vi "RayFanModelIntersection.vi"() -> ()   [LabVIEW 2014]
panel:
  in  "Power":dbl=1200.0 format="%#_13g"
  out "Temp":dbl
  in  "Outside":bool
  out "WeldVsRadius":dbl[](graph)=[1.0, 1.0, 1.0, 1.0, 1.0, 1.0, 1.0, 1.0, 1.0, 1.0, 0.958, 0.93, 0.89, 0.876, 0.852, 0.832, 0.814, 0.8, 0.788, 0.77]
  out "BinSize (mm)":dbl=0.05
  in  "NumBins":dbl=20.0
  out "Dists":cluster{dbl[]}[](array[cluster])=[{[]}, {[]}, {[0.558064432912235]}, {[0.7065110965552522]}, {[]}, {[]}, {[]}, {[]}, {[]}, {[]}, {[]}, {[]}, {[]}, {[]}, {[]}, {[0.5450720152295433]}, {[]}, {[]}, {[]}, {[]}, {[0.7012931044326173]}, {[]}, {[]}, {[]}, {[]}, {[]}, {[]}, {[]}, {[0.7332327965683694]}, {[]}, {[]}, {[]}, {[]}, {[0.9493389374686801]}, {[]}, {[]}, {[]}, {[]}, {[]}, {[]}, {[]}, {[0.64928815624828]}, {[]}, {[0.5406762941256205]}, {[]}, {[]}, {[]}, {[]}, {[]}, {[]}, {[]}, {[]}, {[]}, {[0.5086855573476655]}, {[0.5165368704444614]}, {[]}, {[]}, {[0.9647195737987346]}, {[]}, {[]}, {[]}, {[]}, {[0.6161935056556245]}, {[]}, {[]}, {[]}, {[0.6599666981158043]}, {[0.7575878284267049]}, {[]}, {[]}, {[]}, {[0.6345232898235499]}, {[]}, {[]}, {[0.6975266082013275]}, {[]}, {[0.5491594605386263]}, {[0.5884365935336494]}, {[]}, {[]}, {[0.550418714991808]}, {[]}, {[]}, {[]}, {[]}, {[]}, {[]}, {[]}, {[]}, {[0.547517307123691]}, {[]}, {[]}, {[0.9629712723340546]}, {[]}, {[]}, {[]}, {[]}, {[]}, {[0.7196533645578476]}, {[]}, {[]}, {[0.7873333536260919]}, {[0.5571630383766993]}, {[]}, {[]}, {[]}, {[]}, {[]}, {[]}, {[]}, {[]}, {[]}, {[]}, {[]}, {[]}, {[]}, {[]}, {[]}, {[]}, {[]}, {[0.8921440487629841]}, {[]}, {[]}, {[0.5170623590293416]}, {[0.6003465621820364]}, {[]}, {[]}, {[0.7197465893934318]}, {[]}, {[]}, {[]}, {[]}, {[0.6422717159108584]}, {[]}, {[]}, {[]}, {[]}, {[0.8502006061404428]}, {[]}, {[]}, {[]}, {[]}, {[]}, {[]}, {[]}, {[0.8002135268034918]}, {[]}, {[0.9244653981574149]}, {[]}, {[]}, {[]}, {[]}, {[]}, {[]}, {[0.8127103296432845]}, {[0.8494637102867976]}, {[]}, {[0.5768330500604705]}, {[]}, {[]}, {[0.7971462061943174]}, {[0.5190450538376525]}, {[]}, {[]}, {[0.54203797008764]}, {[]}, {[0.8445112253029017]}, {[]}, {[]}, {[]}, {[]}, {[0.6062550701542475]}, {[]}, {[]}, {[]}, {[]}, {[]}, {[0.7489732042547229]}, {[]}, {[0.8330170817130215]}, {[]}, {[]}, {[]}, {[0.5113666314516164]}, {[0.5498423755123026]}, {[0.7182864687625854]}, {[]}, {[]}, {[]}, {[]}, {[0.6517000534238575]}, {[]}, {[]}, {[0.5789678042492773]}, {[]}, {[]}, {[0.8993049672269428]}, {[0.6085788863115259]}, {[]}, {[0.6204881702091252]}, {[0.9649855049671213]}, {[0.660813864499079]}, {[0.9515616425304806]}, {[]}, {[0.8860520397526913]}, {[]}, {[0.97607827123549]}, {[]}, {[]}, {[]}, {[0.7559538054396471]}, {[]}, {[]}, {[0.8221698352656399]}, {[]}, {[]}, {[]}, {[]}, {[]}, {[]}, {[]}, {[0.5536090969205018]}, {[]}, {[]}, {[]}, {[]}, {[]}, {[0.702817978975694]}, {[]}, {[]}, {[0.6470947342089964]}, {[]}, {[]}, {[0.8120625142610847]}, {[0.5281933009897772]}, {[]}, {[]}, {[]}, {[]}, {[]}, {[]}, {[0.5260646334990027]}, {[]}, {[]}, {[]}, {[]}, {[0.5578229776474865]}, {[]}, {[]}, {[]}, {[]}, {[]}, {[]}, {[]}, {[0.6516324141278934]}, {[]}, {[]}, {[]}, {[0.7277751404296459]}, {[]}, {[0.7346441626947963]}, {[]}, {[0.6018486699053848]}, {[]}, {[]}, {[]}, {[]}, {[0.6609968544557817]}, {[]}, {[]}, {[0.8624857635568423]}, {[]}, {[]}, {[]}, {[]}, {[0.5223973616642758]}, {[]}, {[]}, {[]}, {[]}, {[]}, {[]}, {[]}, {[]}, {[0.6499055476854614]}, {[]}, {[]}, {[]}, {[]}, {[]}, {[]}, {[]}, {[]}, {[]}, {[]}, {[]}, {[]}, {[]}, {[]}, {[]}, {[]}, {[]}, {[]}, {[]}, {[]}, {[]}, {[0.9645688700654612]}, {[]}, {[]}, {[]}, {[]}, {[]}, {[0.8409319062965085]}, {[0.5676961462040259]}, {[0.5428966812044365]}, {[]}, {[]}, {[]}, {[]}, {[]}, {[]}, {[]}, {[]}, {[]}, {[]}, {[0.6075630097775284]}, {[0.6825860604163353]}, {[0.5509754449188999]}, {[0.6287420680195404]}, {[]}, {[0.7824466022421895]}, {[]}, {[]}, {[]}, {[]}, {[]}, {[]}, {[]}, {[]}, {[0.92510946600259]}, {[]}, {[]}, {[]}, {[0.8117899400246639]}, {[0.9767679229503767]}, {[]}, {[]}, {[]}, {[]}, {[]}, {[]}, {[]}, {[]}, {[0.7660735839595996]}, {[]}, {[0.7653390306487524]}, {[]}, {[0.6218747267304856]}, {[0.7980078782480812]}, {[]}, {[]}, {[0.6467511427181266]}, {[]}, {[]}, {[]}, {[]}, {[]}, {[]}, {[]}, {[0.961256735044041]}, {[]}, {[0.5285504192342666]}, {[0.7691150491851212]}, {[]}, {[]}, {[]}, {[]}, {[]}, {[]}, {[]}, {[]}, {[]}, {[]}, {[]}, {[]}, {[]}, {[0.6477695496575054]}, {[]}, {[0.5827289010967698]}, {[]}, {[]}, {[]}, {[0.8661418049454438]}, {[]}, {[]}, {[0.9367031742857802]}, {[]}, {[0.5545590410570911]}, {[]}, {[0.5377050699071217]}, {[]}, {[]}, {[0.7438854029234935]}, {[]}, {[]}, {[]}, {[]}, {[]}, {[]}, {[]}, {[]}, {[0.9431758423974651]}, {[]}, {[]}, {[]}, {[]}, {[]}, {[]}, {[]}, {[]}, {[0.6252002539116622]}, {[]}, {[]}, {[]}, {[]}, {[]}, {[]}, {[]}, {[]}, {[]}, {[]}, {[]}, {[0.52847622764937]}, {[0.6440499209435737]}, {[0.5076983622978631]}, {[]}, {[]}, {[]}, {[]}, {[]}, {[]}, {[]}, {[]}, {[]}, {[]}, {[]}, {[]}, {[]}, {[0.5107329517659359]}, {[]}, {[]}, {[]}, {[]}, {[]}, {[]}, {[]}, {[]}, {[]}, {[]}, {[]}, {[]}, {[]}, {[0.8999320044818604]}, {[]}, {[]}, {[]}, {[]}, {[0.524487828892231]}, {[0.6157343526823348]}, {[]}, {[]}, {[]}, {[0.5775248493157631]}, {[0.633099142329562]}, {[]}, {[]}, {[0.9280184819194474]}, {[]}, {[]}, {[]}, {[]}, {[]}, {[]}, {[]}, {[]}, {[]}, {[0.5746835528787432]}, {[]}, {[0.77311121633859]}, {[]}, {[]}, {[]}, {[]}, {[0.7007929147798608]}, {[]}, {[]}, {[]}, {[0.9727918978336536]}, {[]}, {[]}]
  in  "Length":dbl=1.0 format="%#_13g"
  in  "Rays":u32=500
  in  "Point":cluster{"X":dbl, "Y":dbl, "Z":dbl}={"X"=0.0, "Y"=3.0, "Z"=7.45}
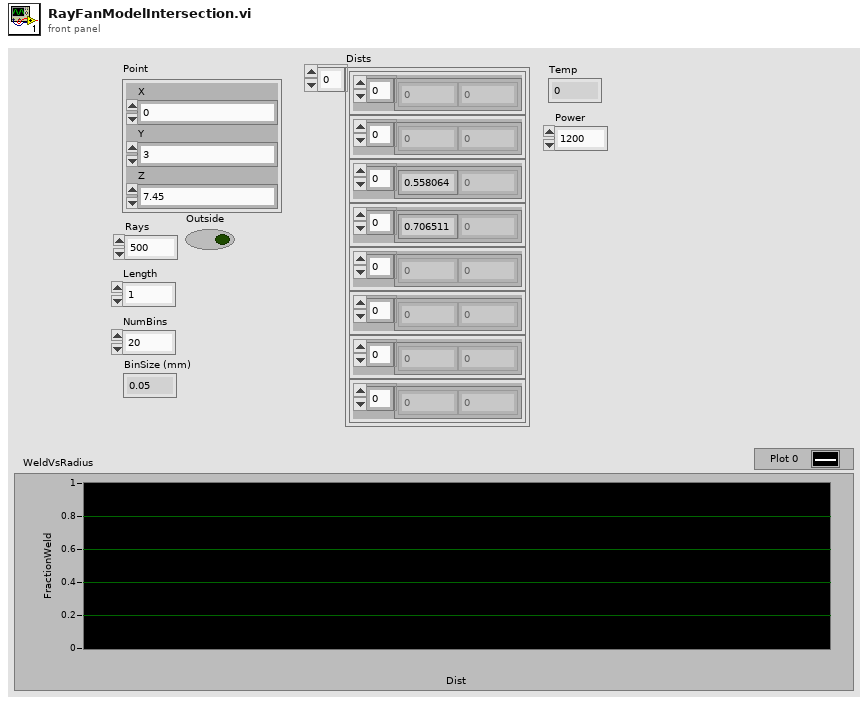
[diagram p1: front panel]
types:
  T1 = cluster{"Point":cluster{"X":dbl, "Y":dbl, "Z":dbl}, cluster{"X":dbl, "Y":dbl, "Z":dbl}}[]
  T2 = typedef "TriangleFace.ctl" = cluster{"Normal":T3, "Vertex1":T3, "Vertex2":T3, "Vertex3":T3}
  T3 = typedef "Point3D.ctl" = cluster{"X":sgl, "Y":sgl, "Z":sgl}
  T4 = cluster{"TriVertex":dbl[][], "Normal":dbl[][], "u":dbl[][], "v":dbl[][]}
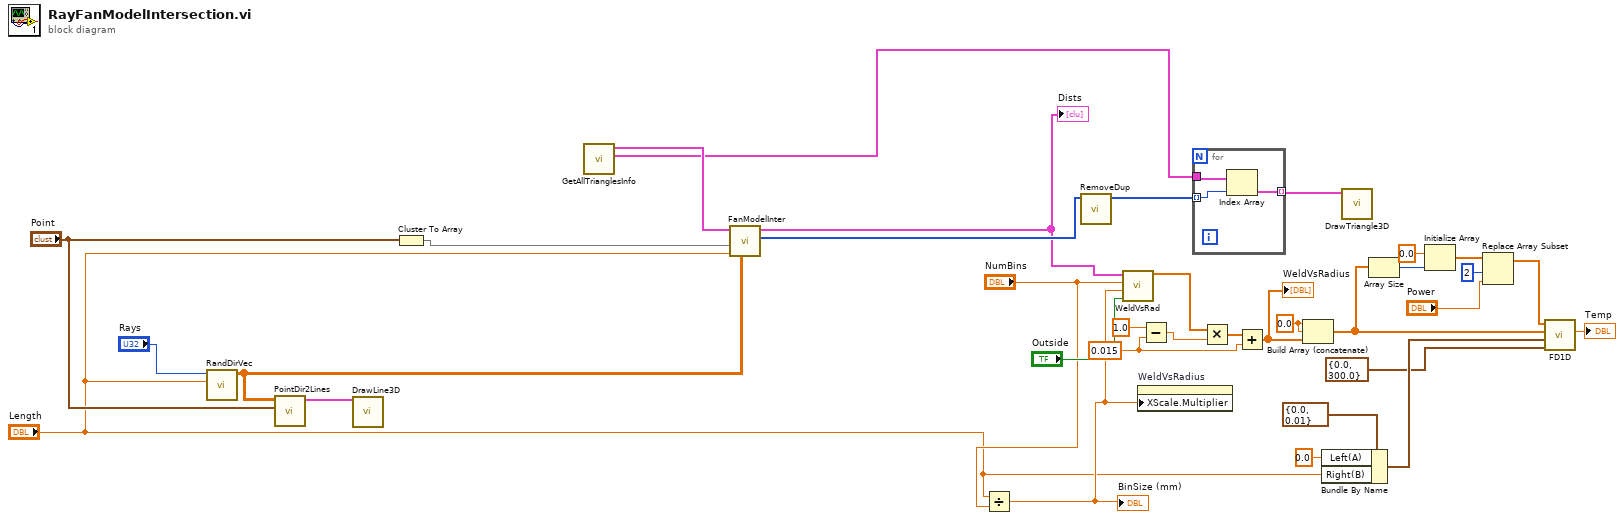
[diagram p0: block diagram]
diagram:
  w2 = 0.015 ("y")
  w20 = 0.0 ("element")
  n1 = call "RandDirVec.vi"("Length"="Length", "Rays"="Rays") -> ("DirVecs"=w30:dbl[][])  [unwired: 9 in]
  n2 = call "PointDir2Lines.vi"("Point"="Point", "DirVecs"=w30) -> ("Lines"=w33:T1)  [unwired: 9 in]
  n3 = call "DrawLine3D.vi"("Lines"=w33) -> ()  [unwired: 11 in]
  n4 = Cluster To Array(cluster="Point") -> (array=w31:dbl[])
  n5 = call "GetAllTrianglesInfo.vi"() -> ("AllTriangles"=w21:T2[], "TriangleInfo"=w22:T4)  [unwired: 10 in]
  n6 = call "FanModelInter.vi"("DirVecs"=w30, "Length"="Length", "Point"=w31, "TriangleInfo"=w22) -> ("TriangleIndexes"=w29:i32[], "Dists"=w26:cluster{dbl[]}[])  [unwired: 6 in]
  "Dists" <- w26
  n7 = Divide(x="Length", y="NumBins") -> (x/y=w23:dbl)
  "BinSize (mm)" <- w23
  n8 = call "RemoveDup.vi"("Index"=w29) -> ("DupRemoved"=w28:i32[])  [unwired: 10 in]
  n9 = call "WeldVsRad.vi"("Outside"="Outside", "BinSize (mm)"=w23, "NumBins"="NumBins", "Dists"=w26) -> ("WeldVsRadius"=w6:dbl[])  [unwired: 7 in]
  n10 = property on="WeldVsRadius" class="WFGraph (strict)"("XScale.Multiplier"=w23) -> ()  [unwired: 2 in, 2 out]
  n11 = Subtract(x=1.0, y=w2) -> (x-y=w4:dbl)
  n12 = for {
    tunnel: w21 -> [w36]
    tunnel: w28 -> [w37] mode=indexing
    tunnel: [w35] -> w27 mode=indexing
    n13 = Index Array(array=w36, index=w37) -> (element=w35:T2)
  }
  n14 = Multiply(x=w6, y=w4) -> (x*y=w3:dbl[])
  n15 = Add(x=w3, y=w2) -> (x+y=w1:dbl[])
  "WeldVsRadius" <- w1
  n16 = Build Array (concatenate)(w20, w20, w1) -> (w14:dbl[])
  n17 = Bundle By Name(cluster=cluster{"Left(A)":dbl, "Right(B)":dbl} {"Left(A)"=0.0, "Right(B)"=0.01} ("Xendpoints"), "Left(A)"=0.0, "Right(B)"="Length") -> (w16:cluster{"Left(A)":dbl, "Right(B)":dbl})
  n18 = call "DrawTriangle3D.vi"("Triangles"=w27) -> ()  [unwired: 11 in]
  n19 = Array Size(array=w14) -> (size(s)=w13:i32)
  n20 = Initialize Array(0.0 ("element"), w13) -> (w11:dbl[])
  n21 = Replace Array Subset(array=w11, new element="Power", index=2) -> (w8:dbl[])
  n22 = call "FD1D.vi"("Temps"=cluster{"Left(UA)":dbl, "Right(UB)":dbl} {"Left(UA)"=0.0, "Right(UB)"=300.0}, "Xendpoints"=w16, "K"=w14, "F"=w8) -> ("Temp"=→"Temp":dbl)  [unwired: 6 in, 1 out]
